vi "Laundry Machine.vi"() -> ()   [LabVIEW 2011]
panel:
  out "1-Rinsing\n2-Washing\n3-Squeezing\n4-Drying":i16[](array[numeric])
  in  "?":bool
  in  "?":bool
  in  "?":bool
  in  "?":bool
  in  "?":bool
  in  "Washing Time(1)":dbl
  in  "Drying Time":dbl
  in  "Squeezing Time":dbl
  in  "Washing Time(2)":dbl
  in  "Rinsing Time":dbl
  in  "Air Temp Variation":dbl
  out "Air Temperature":dbl(slide) scale=0.0..100.0
  out "Air Comp On":bool
  out "Resistor On":bool
  in  "Initial Water Temperature":dbl
  out "Filthy Water":dbl(slide) scale=0.0..10.0
  out "RPM":dbl(knob) scale=0.0..60.0
  out "Mass Flow Rate":dbl(knob) scale=0.0..40.0
  in  "Soap(g)":dbl(slide) scale=0.0..1000.0
  in  "Set Water Temperature":i8(knob) scale=20.0..100.0
  out "Water Temperature(C)":i8(slide) scale=0.0..100.0
  in  "Tank(L)":dbl(slide) scale=0.0..10.0
  in  "Weight":u8
  out "Door Locked":bool
  in  "Lock Door":bool
  in  "Program":i8(knob) scale=0.0..3.0
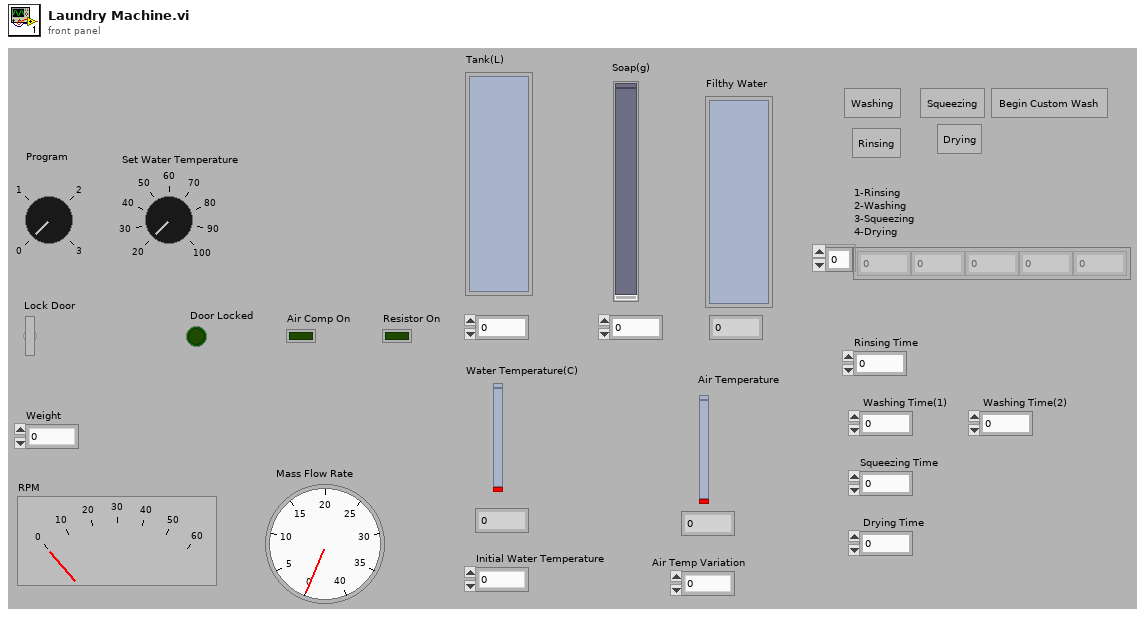
[diagram p1: front panel]
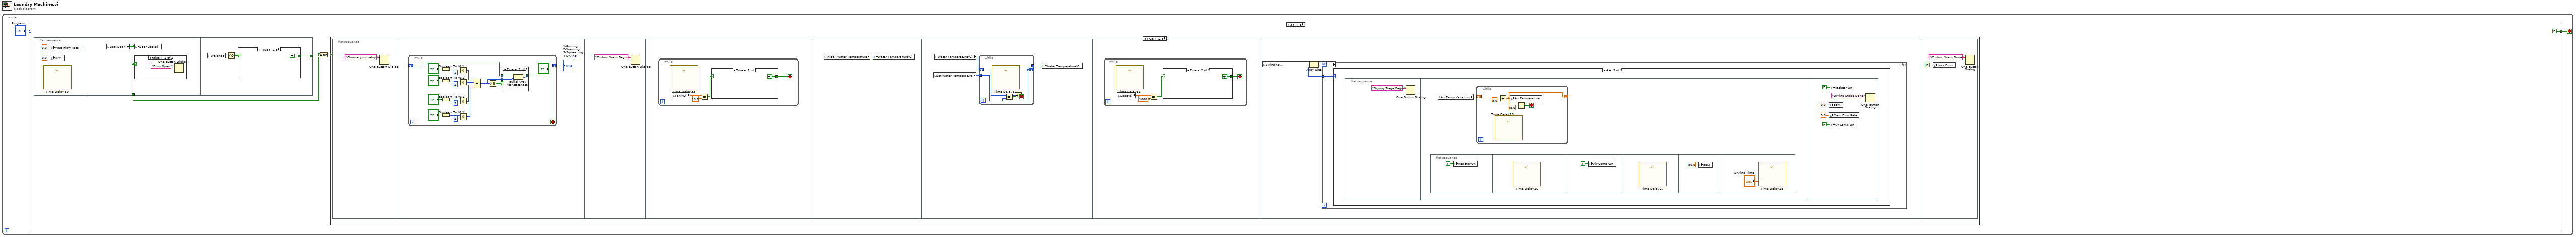
[diagram p0: block diagram]
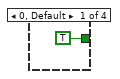
[diagram p2: hidden frame]
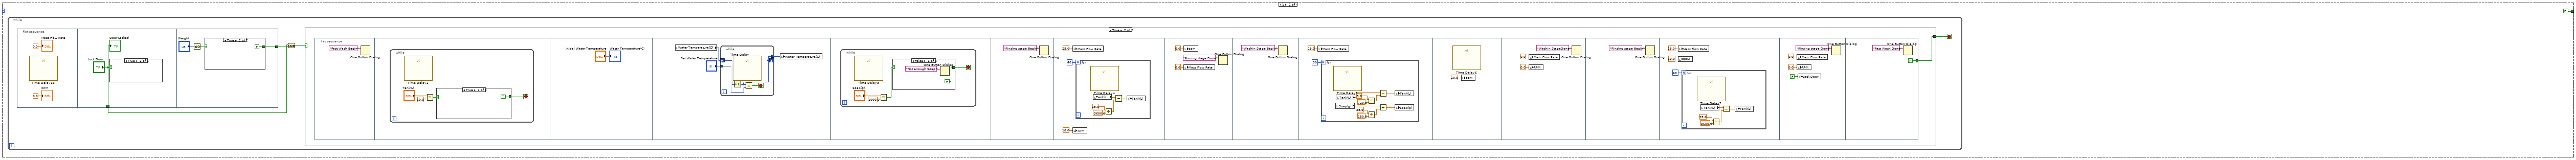
[diagram p3: hidden frame]
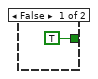
[diagram p4: hidden frame]
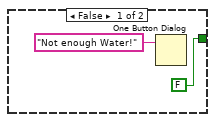
[diagram p5: hidden frame]
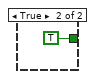
[diagram p6: hidden frame]
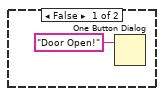
[diagram p7: hidden frame]
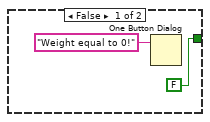
[diagram p8: hidden frame]
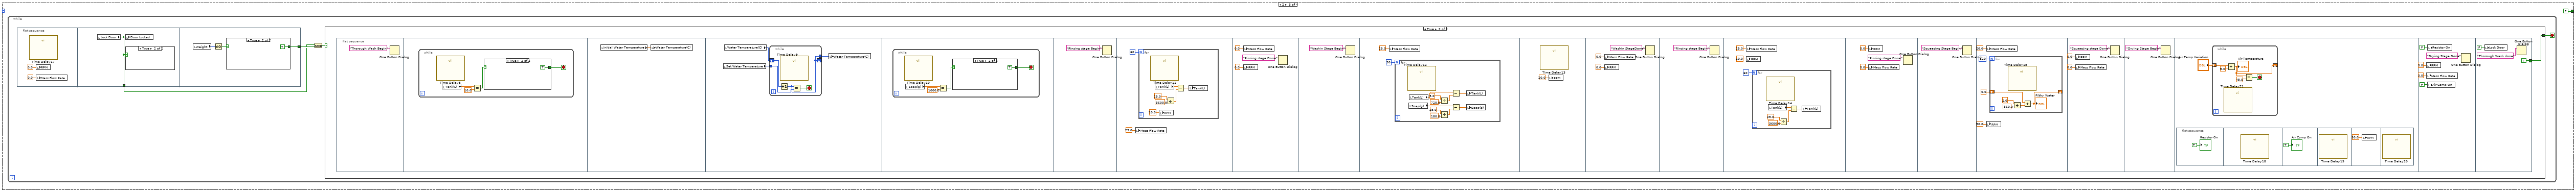
[diagram p9: hidden frame]
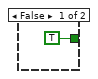
[diagram p10: hidden frame]
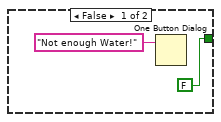
[diagram p11: hidden frame]
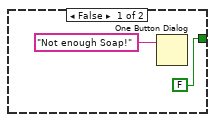
[diagram p12: hidden frame]
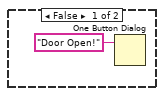
[diagram p13: hidden frame]
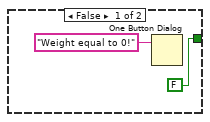
[diagram p14: hidden frame]
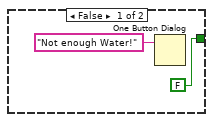
[diagram p17: hidden frame]
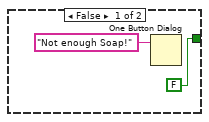
[diagram p18: hidden frame]
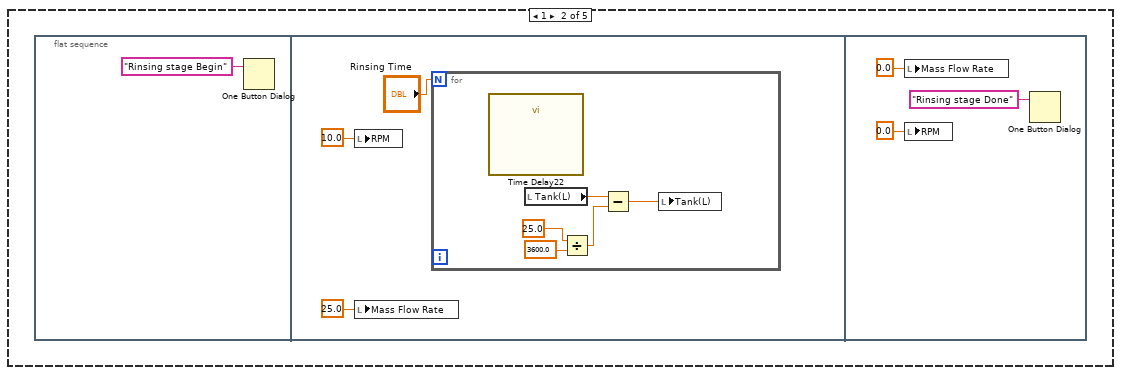
[diagram p20: hidden frame]
diagram:
  n1 = while {
    stop <- w2 stop-if-true
    n2 = case shown="3" "Program" {
      tunnel: [TRUE FALSE FALSE FALSE] -> w2
      frame 0, Default {
      }
      frame 1 {
        n3 = while {
          stop <- w5 stop-if-true
          n4 = flat-sequence {
            tunnel: ["Lock Door"] -> w8
            tunnel: [w82] -> w7
            frame #0 {
              n5 = call "Time Delay16"() -> ()  [unwired: 11 in, 1 out]
              "Mass Flow Rate" <- 0.0 ("Mass Flow Rate")
              "RPM" <- 0.0 ("RPM")
            }
            frame #1 {
              n6 = case shown="True" "Lock Door" {
                frame False {
                  n7 = One Button Dialog(message="Door Open!") -> ()  [unwired: 1 in, 1 out]
                }
                frame True {
                }
              }
              "Door Locked" <- "Lock Door"
            }
            frame #2 {
              n8 = Not Equal To 0?(x="Weight") -> (x != 0?=w83:bool)
              n9 = case shown="True" w83 {
                tunnel: [FALSE TRUE] -> w82
                frame False {
                  n10 = One Button Dialog(message="Weight equal to 0!") -> ()  [unwired: 1 in, 1 out]
                }
                frame True {
                }
              }
            }
          }
          n11 = And(x=w8, y=w7) -> (x .and. y?=w6:bool)
          n12 = case shown="True" w6 {
            tunnel: [TRUE w10] -> w5
            frame False {
            }
            frame True {
              n13 = flat-sequence {
                tunnel: [TRUE] -> w10
                frame #0 {
                  n14 = One Button Dialog(message="Fast Wash Begin" ("Stage")) -> ()  [unwired: 1 in, 1 out]
                }
                frame #1 {
                  n15 = while {
                    stop <- w13 stop-if-true
                    n16 = call "Time Delay2"() -> ()  [unwired: 11 in, 1 out]
                    n17 = Equal?(x="Tank(L)", y=10.0) -> (x = y?=w14:bool)
                    n18 = case shown="True" w14 {
                      tunnel: [FALSE TRUE] -> w13
                      frame False {
                        n19 = One Button Dialog(message="Not enough Water!" ("String 2")) -> ()  [unwired: 1 in, 1 out]
                      }
                      frame True {
                      }
                    }
                  }
                }
                frame #2 {
                  "Water Temperature(C)" <- "Initial Water Temperature"
                }
                frame #3 {
                  n20 = local read "Water Temperature(C)"() -> (w21:i8)
                  n21 = while {
                    tunnel: "Set Water Temperature" -> [w26]
                    shift-right: [w23] -> _
                    shift-left: w21 -> [w24]
                    tunnel: [w23] -> w20
                    stop <- w25 stop-if-true
                    n22 = Increment(x=w24) -> (x+1=w23:i8)
                    n23 = call "Time Delay"() -> ()  [unwired: 11 in, 1 out]
                    n24 = Equal?(x=w23, y=w26) -> (x = y?=w25:bool)
                  }
                  n25 = local write "Water Temperature(C)"(w20) -> ()
                }
                frame #4 {
                  n26 = while {
                    stop <- w28 stop-if-true
                    n27 = call "Time Delay3"() -> ()  [unwired: 11 in, 1 out]
                    n28 = Equal?(x="Soap(g)", y=1000.0) -> (x = y?=w29:bool)
                    n29 = case shown="False" w29 {
                      tunnel: [FALSE TRUE] -> w28
                      frame False {
                        n30 = One Button Dialog(message="Not enough Soap!" ("String 2")) -> ()  [unwired: 1 in, 1 out]
                      }
                      frame True {
                      }
                    }
                  }
                }
                frame #5 {
                  n31 = One Button Dialog(message="Rinsing stage Begin" ("Stage")) -> ()  [unwired: 1 in, 1 out]
                }
                frame #6 {
                  n32 = local write "Mass Flow Rate"(25.0 ("Mass Flow Rate")) -> ()
                  n33 = local write "RPM"(10.0 ("RPM")) -> ()
                  n34 = for {
                    N: 60 -> [_]
                    n35 = call "Time Delay4"() -> ()  [unwired: 11 in, 1 out]
                    n36 = local read "Tank(L)"() -> (w38:dbl)
                    n37 = Divide(x=25.0, y=3600.0) -> (x/y=w40:dbl)
                    n38 = Subtract(x=w38, y=w40) -> (x-y=w39:dbl)
                    n39 = local write "Tank(L)"(w39) -> ()
                  }
                }
                frame #7 {
                  n40 = local write "RPM"(0.0 ("RPM")) -> ()
                  n41 = local write "Mass Flow Rate"(0.0 ("Mass Flow Rate")) -> ()
                  n42 = One Button Dialog(message="Rinsing stage Done" ("Stage")) -> ()  [unwired: 1 in, 1 out]
                }
                frame #8 {
                  n43 = One Button Dialog(message="Washin Stage Begin" ("Stage")) -> ()  [unwired: 1 in, 1 out]
                }
                frame #9 {
                  n44 = local write "Mass Flow Rate"(25.0 ("Mass Flow Rate")) -> ()
                  n45 = for {
                    N: 30 -> [_]
                    n46 = call "Time Delay5"() -> ()  [unwired: 11 in, 1 out]
                    n47 = local read "Soap(g)"() -> (w57:dbl)
                    n48 = local read "Tank(L)"() -> (w50:dbl)
                    n49 = Divide(x=5.0, y=720.0) -> (x/y=w52:dbl)
                    n50 = Divide(x=25.0, y=180.0) -> (x/y=w56:dbl)
                    n51 = Subtract(x=w50, y=w52) -> (x-y=w53:dbl)
                    n52 = Subtract(x=w57, y=w56) -> (x-y=w58:dbl)
                    n53 = local write "Tank(L)"(w53) -> ()
                    n54 = local write "Soap(g)"(w58) -> ()
                  }
                }
                frame #10 {
                  n55 = call "Time Delay6"() -> ()  [unwired: 11 in, 1 out]
                  n56 = local write "RPM"(20.0 ("RPM")) -> ()
                }
                frame #11 {
                  n57 = local write "Mass Flow Rate"(0.0 ("Mass Flow Rate")) -> ()
                  n58 = local write "RPM"(0.0 ("RPM")) -> ()
                  n59 = One Button Dialog(message="Washin StageDone" ("Stage")) -> ()  [unwired: 1 in, 1 out]
                }
                frame #12 {
                  n60 = One Button Dialog(message="Rinsing stage Begin" ("Stage")) -> ()  [unwired: 1 in, 1 out]
                }
                frame #13 {
                  n61 = local write "Mass Flow Rate"(25.0 ("Mass Flow Rate")) -> ()
                  n62 = local write "RPM"(10.0 ("RPM")) -> ()
                  n63 = for {
                    N: 60 -> [_]
                    n64 = call "Time Delay7"() -> ()  [unwired: 11 in, 1 out]
                    n65 = local read "Tank(L)"() -> (w67:dbl)
                    n66 = Divide(x=25.0, y=3600.0) -> (x/y=w69:dbl)
                    n67 = Subtract(x=w67, y=w69) -> (x-y=w68:dbl)
                    n68 = local write "Tank(L)"(w68) -> ()
                  }
                }
                frame #14 {
                  n69 = local write "Mass Flow Rate"(0.0 ("Mass Flow Rate")) -> ()
                  n70 = local write "RPM"(0.0 ("RPM")) -> ()
                  n71 = local write "Lock Door"(FALSE ("Lock Door")) -> ()
                  n72 = One Button Dialog(message="Rinsing stage Done" ("Stage")) -> ()  [unwired: 1 in, 1 out]
                }
                frame #15 {
                  n73 = One Button Dialog(message="Fast Wash Done" ("Stage")) -> ()  [unwired: 1 in, 1 out]
                }
              }
            }
          }
        }
      }
      frame 2 {
        n74 = while {
          stop <- w90 stop-if-true
          n75 = flat-sequence {
            tunnel: [w192] -> w89
            tunnel: [w195] -> w92
            frame #0 {
              n76 = call "Time Delay17"() -> ()  [unwired: 11 in, 1 out]
              n77 = local write "RPM"(0.0 ("RPM")) -> ()
              n78 = local write "Mass Flow Rate"(0.0 ("Mass Flow Rate")) -> ()
            }
            frame #1 {
              n79 = local read "Lock Door"() -> (w192:bool)
              n80 = local write "Door Locked"(w192) -> ()
              n81 = case shown="True" w192 {
                frame False {
                  n82 = One Button Dialog(message="Door Open!") -> ()  [unwired: 1 in, 1 out]
                }
                frame True {
                }
              }
            }
            frame #2 {
              n83 = local read "Weight"() -> (w194:u8)
              n84 = Not Equal To 0?(x=w194) -> (x != 0?=w196:bool)
              n85 = case shown="True" w196 {
                tunnel: [FALSE TRUE] -> w195
                frame False {
                  n86 = One Button Dialog(message="Weight equal to 0!") -> ()  [unwired: 1 in, 1 out]
                }
                frame True {
                }
              }
            }
          }
          n87 = And(x=w89, y=w92) -> (x .and. y?=w91:bool)
          n88 = case shown="True" w91 {
            tunnel: [TRUE w94] -> w90
            frame False {
            }
            frame True {
              n89 = flat-sequence {
                tunnel: [TRUE] -> w94
                frame #0 {
                  n90 = One Button Dialog(message="Thorough Wash Begin" ("Stage")) -> ()  [unwired: 1 in, 1 out]
                }
                frame #1 {
                  n91 = while {
                    stop <- w97 stop-if-true
                    n92 = call "Time Delay8"() -> ()  [unwired: 11 in, 1 out]
                    n93 = local read "Tank(L)"() -> (w96:dbl)
                    n94 = Equal?(x=w96, y=10.0) -> (x = y?=w98:bool)
                    n95 = case shown="True" w98 {
                      tunnel: [FALSE TRUE] -> w97
                      frame False {
                        n96 = One Button Dialog(message="Not enough Water!" ("String 2")) -> ()  [unwired: 1 in, 1 out]
                      }
                      frame True {
                      }
                    }
                  }
                }
                frame #2 {
                  n97 = local read "Initial Water Temperature"() -> (w103:dbl)
                  n98 = local write "Water Temperature(C)"(w103) -> ()
                }
                frame #3 {
                  n99 = local read "Set Water Temperature"() -> (w105:i8)
                  n100 = local read "Water Temperature(C)"() -> (w106:i8)
                  n101 = while {
                    tunnel: w105 -> [w110]
                    shift-right: [w107] -> _
                    shift-left: w106 -> [w108]
                    tunnel: [w107] -> w104
                    stop <- w109 stop-if-true
                    n102 = Increment(x=w108) -> (x+1=w107:i8)
                    n103 = call "Time Delay9"() -> ()  [unwired: 11 in, 1 out]
                    n104 = Equal?(x=w107, y=w110) -> (x = y?=w109:bool)
                  }
                  n105 = local write "Water Temperature(C)"(w104) -> ()
                }
                frame #4 {
                  n106 = while {
                    stop <- w112 stop-if-true
                    n107 = call "Time Delay10"() -> ()  [unwired: 11 in, 1 out]
                    n108 = local read "Soap(g)"() -> (w111:dbl)
                    n109 = Equal?(x=w111, y=1000.0) -> (x = y?=w113:bool)
                    n110 = case shown="True" w113 {
                      tunnel: [FALSE TRUE] -> w112
                      frame False {
                        n111 = One Button Dialog(message="Not enough Soap!" ("String 2")) -> ()  [unwired: 1 in, 1 out]
                      }
                      frame True {
                      }
                    }
                  }
                }
                frame #5 {
                  n112 = One Button Dialog(message="Rinsing stage Begin" ("Stage")) -> ()  [unwired: 1 in, 1 out]
                }
                frame #6 {
                  n113 = local write "Mass Flow Rate"(25.0 ("Mass Flow Rate")) -> ()
                  n114 = for {
                    N: 60 -> [_]
                    n115 = call "Time Delay11"() -> ()  [unwired: 11 in, 1 out]
                    n116 = local read "Tank(L)"() -> (w124:dbl)
                    n117 = local write "RPM"(10.0 ("RPM")) -> ()
                    n118 = Divide(x=25.0, y=3600.0) -> (x/y=w123:dbl)
                    n119 = Subtract(x=w124, y=w123) -> (x-y=w125:dbl)
                    n120 = local write "Tank(L)"(w125) -> ()
                  }
                }
                frame #7 {
                  n121 = local write "Mass Flow Rate"(0.0 ("RPM")) -> ()
                  n122 = local write "RPM"(0.0 ("Mass Flow Rate")) -> ()
                  n123 = One Button Dialog(message="Rinsing stage Done" ("Stage")) -> ()  [unwired: 1 in, 1 out]
                }
                frame #8 {
                  n124 = One Button Dialog(message="Washin Stage Begin" ("Stage")) -> ()  [unwired: 1 in, 1 out]
                }
                frame #9 {
                  n125 = local write "Mass Flow Rate"(25.0 ("Mass Flow Rate")) -> ()
                  n126 = for {
                    N: 30 -> [_]
                    n127 = call "Time Delay12"() -> ()  [unwired: 11 in, 1 out]
                    n128 = local read "Soap(g)"() -> (w139:dbl)
                    n129 = local read "Tank(L)"() -> (w141:dbl)
                    n130 = Divide(x=5.0, y=720.0) -> (x/y=w135:dbl)
                    n131 = Divide(x=25.0, y=180.0) -> (x/y=w138:dbl)
                    n132 = Subtract(x=w141, y=w135) -> (x-y=w142:dbl)
                    n133 = Subtract(x=w139, y=w138) -> (x-y=w140:dbl)
                    n134 = local write "Tank(L)"(w142) -> ()
                    n135 = local write "Soap(g)"(w140) -> ()
                  }
                }
                frame #10 {
                  n136 = call "Time Delay13"() -> ()  [unwired: 11 in, 1 out]
                  n137 = local write "RPM"(20.0 ("RPM")) -> ()
                }
                frame #11 {
                  n138 = local write "Mass Flow Rate"(0.0 ("Mass Flow Rate")) -> ()
                  n139 = local write "RPM"(0.0 ("RPM")) -> ()
                  n140 = One Button Dialog(message="Washin StageDone" ("Stage")) -> ()  [unwired: 1 in, 1 out]
                }
                frame #12 {
                  n141 = One Button Dialog(message="Rinsing stage Begin" ("Stage")) -> ()  [unwired: 1 in, 1 out]
                }
                frame #13 {
                  n142 = local write "Mass Flow Rate"(25.0 ("Mass Flow Rate")) -> ()
                  n143 = local write "RPM"(10.0 ("RPM")) -> ()
                  n144 = for {
                    N: 60 -> [_]
                    n145 = call "Time Delay14"() -> ()  [unwired: 11 in, 1 out]
                    n146 = local read "Tank(L)"() -> (w151:dbl)
                    n147 = Divide(x=25.0, y=3600.0) -> (x/y=w153:dbl)
                    n148 = Subtract(x=w151, y=w153) -> (x-y=w152:dbl)
                    n149 = local write "Tank(L)"(w152) -> ()
                  }
                }
                frame #14 {
                  n150 = local write "RPM"(0.0 ("RPM")) -> ()
                  n151 = local write "Mass Flow Rate"(0.0 ("Mass Flow Rate")) -> ()
                  n152 = One Button Dialog(message="Rinsing stage Done" ("Stage")) -> ()  [unwired: 1 in, 1 out]
                }
                frame #15 {
                  n153 = One Button Dialog(message="Squeezing Stage Begin" ("Stage")) -> ()  [unwired: 1 in, 1 out]
                }
                frame #16 {
                  n154 = local write "Mass Flow Rate"(20.0 ("Mass Flow Rate")) -> ()
                  n155 = local write "RPM"(50.0 ("RPM")) -> ()
                  n156 = for {
                    N: 120 -> [_]
                    shift-right: [w164] -> _
                    shift-left: 0.0 -> [w165]
                    n157 = call "Time Delay15"() -> ()  [unwired: 11 in, 1 out]
                    n158 = Divide(x=2.0, y=360.0) -> (x/y=w166:dbl)
                    n159 = Add(x=w165, y=w166) -> (x+y=w164:dbl)
                    "Filthy Water" <- w164
                  }
                }
                frame #17 {
                  n160 = local write "RPM"(0.0 ("RPM")) -> ()
                  n161 = local write "Mass Flow Rate"(0.0 ("Mass Flow Rate")) -> ()
                  n162 = One Button Dialog(message="Squeezing stage Done" ("Stage")) -> ()  [unwired: 1 in, 1 out]
                }
                frame #18 {
                  n163 = One Button Dialog(message="Drying Stage Begin" ("Stage")) -> ()  [unwired: 1 in, 1 out]
                }
                frame #19 {
                  n164 = flat-sequence {
                    frame #0 {
                      "Resistor On" <- TRUE ("Resistor On")
                    }
                    frame #1 {
                      n165 = call "Time Delay18"() -> ()  [unwired: 11 in, 1 out]
                    }
                    frame #2 {
                      "Air Comp On" <- TRUE ("Air Comp On")
                    }
                    frame #3 {
                      n166 = call "Time Delay19"() -> ()  [unwired: 11 in, 1 out]
                    }
                    frame #4 {
                      n167 = local write "RPM"(50.0 ("RPM")) -> ()
                    }
                    frame #5 {
                      n168 = call "Time Delay20"() -> ()  [unwired: 11 in, 1 out]
                    }
                  }
                  n169 = while {
                    shift-right: [w175] -> _
                    shift-left: "Air Temp Variation" -> [w174]
                    stop <- w176 stop-if-true
                    n170 = call "Time Delay21"() -> ()  [unwired: 11 in, 1 out]
                    n171 = Add(x=w174, y=5.0) -> (x+y=w175:dbl)
                    "Air Temperature" <- w175
                    n172 = Equal?(x=w175, y=45.0) -> (x = y?=w176:bool)
                  }
                }
                frame #20 {
                  n173 = local write "RPM"(0.0 ("RPM")) -> ()
                  n174 = local write "Mass Flow Rate"(0.0 ("Mass Flow Rate")) -> ()
                  n175 = local write "Resistor On"(FALSE ("Resistor On")) -> ()
                  n176 = local write "Air Comp On"(FALSE ("Air Comp On")) -> ()
                  n177 = One Button Dialog(message="Drying Stage Done" ("Stage")) -> ()  [unwired: 1 in, 1 out]
                }
                frame #21 {
                  n178 = local write "Lock Door"(FALSE ("Lock Door")) -> ()
                  n179 = One Button Dialog(message="Thorough Wash done" ("Stage")) -> ()  [unwired: 1 in, 1 out]
                }
              }
            }
          }
        }
      }
      frame 3 {
        n180 = flat-sequence {
          tunnel: [w320] -> w201
          tunnel: [w323] -> w202
          frame #0 {
            n181 = call "Time Delay30"() -> ()  [unwired: 11 in, 1 out]
            n182 = local write "Mass Flow Rate"(0.0 ("Mass Flow Rate")) -> ()
            n183 = local write "RPM"(0.0 ("RPM")) -> ()
          }
          frame #1 {
            n184 = local read "Lock Door"() -> (w320:bool)
            n185 = local write "Door Locked"(w320) -> ()
            n186 = case shown="False" w320 {
              frame False {
                n187 = One Button Dialog(message="Door Open!") -> ()  [unwired: 1 in, 1 out]
              }
              frame True {
              }
            }
          }
          frame #2 {
            n188 = local read "Weight"() -> (w322:u8)
            n189 = Not Equal To 0?(x=w322) -> (x != 0?=w324:bool)
            n190 = case shown="True" w324 {
              tunnel: [FALSE TRUE] -> w323
              frame False {
                n191 = One Button Dialog(message="Weight equal to 0!") -> ()  [unwired: 1 in, 1 out]
              }
              frame True {
              }
            }
          }
        }
        n192 = And(x=w201, y=w202) -> (x .and. y?=w200:bool)
        n193 = case shown="True" w200 {
          frame False {
          }
          frame True {
            n194 = flat-sequence {
              frame #0 {
                n195 = One Button Dialog(message="Choose your setup" ("Stage")) -> ()  [unwired: 1 in, 1 out]
              }
              frame #1 {
                n196 = while {
                  shift-right: [w208] -> w205
                  shift-left: _ -> [w206]
                  stop <- "?" stop-if-true
                  n197 = Boolean To (0,1)(Boolean="?") -> (0, 1=w221:i16)
                  n198 = Boolean To (0,1)(Boolean="?") -> (0, 1=w218:i16)
                  n199 = Boolean To (0,1)(Boolean="?") -> (0, 1=w220:i16)
                  n200 = Boolean To (0,1)(Boolean="?") -> (0, 1=w219:i16)
                  n201 = Multiply(x=w221, y=i16 1) -> (x*y=w213:i16)
                  n202 = Multiply(x=w218, y=i16 2) -> (x*y=w212:i16)
                  n203 = Multiply(x=w220, y=i16 3) -> (x*y=w211:i16)
                  n204 = Multiply(x=w219, y=i16 4) -> (x*y=w210:i16)
                  n205 = Compound Arithmetic op=ADD(w213, w212, w211, w210) -> (w207:i16)
                  n206 = Not Equal To 0?(x=w207) -> (x != 0?=w209:bool)
                  n207 = case shown="True" w209 {
                    tunnel: [w227 w230] -> w208
                    tunnel: w207 -> [_ w229]
                    tunnel: w206 -> [w227 w228]
                    frame False {
                    }
                    frame True {
                      n208 = Build Array (concatenate)(w228, w229) -> (w230:i16[])
                    }
                  }
                }
                "1-Rinsing\n2-Washing\n3-Squeezing\n4-Drying" <- w205
              }
              frame #2 {
                n209 = One Button Dialog(message="Custom Wash Begin" ("Stage")) -> ()  [unwired: 1 in, 1 out]
              }
              frame #3 {
                n210 = while {
                  stop <- w233 stop-if-true
                  n211 = call "Time Delay33"() -> ()  [unwired: 11 in, 1 out]
                  n212 = local read "Tank(L)"() -> (w232:dbl)
                  n213 = Equal?(x=w232, y=10.0) -> (x = y?=w234:bool)
                  n214 = case shown="True" w234 {
                    tunnel: [FALSE TRUE] -> w233
                    frame False {
                      n215 = One Button Dialog(message="Not enough Water!" ("String 2")) -> ()  [unwired: 1 in, 1 out]
                    }
                    frame True {
                    }
                  }
                }
              }
              frame #4 {
                n216 = local read "Initial Water Temperature"() -> (w239:dbl)
                n217 = local write "Water Temperature(C)"(w239) -> ()
              }
              frame #5 {
                n218 = local read "Set Water Temperature"() -> (w241:i8)
                n219 = local read "Water Temperature(C)"() -> (w240:i8)
                n220 = while {
                  tunnel: w241 -> [w246]
                  shift-right: [w243] -> _
                  shift-left: w240 -> [w244]
                  tunnel: [w243] -> w242
                  stop <- w245 stop-if-true
                  n221 = call "Time Delay32"() -> ()  [unwired: 11 in, 1 out]
                  n222 = Increment(x=w244) -> (x+1=w243:i8)
                  n223 = Equal?(x=w243, y=w246) -> (x = y?=w245:bool)
                }
                n224 = local write "Water Temperature(C)"(w242) -> ()
              }
              frame #6 {
                n225 = while {
                  stop <- w248 stop-if-true
                  n226 = call "Time Delay31"() -> ()  [unwired: 11 in, 1 out]
                  n227 = local read "Soap(g)"() -> (w247:dbl)
                  n228 = Equal?(x=w247, y=1000.0) -> (x = y?=w249:bool)
                  n229 = case shown="True" w249 {
                    tunnel: [FALSE TRUE] -> w248
                    frame False {
                      n230 = One Button Dialog(message="Not enough Soap!" ("String 2")) -> ()  [unwired: 1 in, 1 out]
                    }
                    frame True {
                    }
                  }
                }
              }
              frame #7 {
                n231 = local read "1-Rinsing\n2-Washing\n3-Squeezing\n4-Drying"() -> (w254:i16[])
                n232 = Array Size(array=w254) -> (size(s)=w255:i32)
                n233 = for {
                  N: w255 -> [_]
                  tunnel: w254 -> [w256] mode=indexing
                  n234 = case shown="4" w256 {
                    frame 0, Default {
                    }
                    frame 1 {
                      n235 = flat-sequence {
                        frame #0 {
                          n236 = One Button Dialog(message="Rinsing stage Begin" ("Stage")) -> ()  [unwired: 1 in, 1 out]
                        }
                        frame #1 {
                          n237 = local write "RPM"(10.0 ("RPM")) -> ()
                          n238 = local write "Mass Flow Rate"(25.0 ("Mass Flow Rate")) -> ()
                          n239 = for {
                            N: "Rinsing Time" -> [_]
                            n240 = call "Time Delay22"() -> ()  [unwired: 11 in, 1 out]
                            n241 = local read "Tank(L)"() -> (w264:dbl)
                            n242 = Divide(x=25.0, y=3600.0) -> (x/y=w263:dbl)
                            n243 = Subtract(x=w264, y=w263) -> (x-y=w265:dbl)
                            n244 = local write "Tank(L)"(w265) -> ()
                          }
                        }
                        frame #2 {
                          n245 = local write "Mass Flow Rate"(0.0 ("RPM")) -> ()
                          n246 = local write "RPM"(0.0 ("Mass Flow Rate")) -> ()
                          n247 = One Button Dialog(message="Rinsing stage Done" ("Stage")) -> ()  [unwired: 1 in, 1 out]
                        }
                      }
                    }
                    frame 2 {
                      n248 = flat-sequence {
                        frame #0 {
                          n249 = One Button Dialog(message="Washin Stage Begin" ("Stage")) -> ()  [unwired: 1 in, 1 out]
                        }
                        frame #1 {
                          n250 = local write "Mass Flow Rate"(25.0 ("Mass Flow Rate")) -> ()
                          n251 = for {
                            N: "Washing Time(1)" -> [_]
                            n252 = call "Time Delay24"() -> ()  [unwired: 11 in, 1 out]
                            n253 = local read "Soap(g)"() -> (w278:dbl)
                            n254 = local read "Tank(L)"() -> (w280:dbl)
                            n255 = Divide(x=5.0, y=720.0) -> (x/y=w274:dbl)
                            n256 = Divide(x=25.0, y=180.0) -> (x/y=w277:dbl)
                            n257 = Subtract(x=w280, y=w274) -> (x-y=w281:dbl)
                            n258 = Subtract(x=w278, y=w277) -> (x-y=w279:dbl)
                            n259 = local write "Tank(L)"(w281) -> ()
                            n260 = local write "Soap(g)"(w279) -> ()
                          }
                        }
                        frame #2 {
                          n261 = local write "RPM"(20.0 ("RPM")) -> ()
                          n262 = call "Time Delay23"("Delay Time (s)"="Washing Time(2)") -> ()  [unwired: 10 in, 1 out]
                        }
                        frame #3 {
                          n263 = local write "Mass Flow Rate"(0.0 ("Mass Flow Rate")) -> ()
                          n264 = local write "RPM"(0.0 ("RPM")) -> ()
                          n265 = One Button Dialog(message="Washin StageDone" ("Stage")) -> ()  [unwired: 1 in, 1 out]
                        }
                      }
                    }
                    frame 3 {
                      n266 = flat-sequence {
                        frame #0 {
                          n267 = One Button Dialog(message="Squeezing Stage Begin" ("Stage")) -> ()  [unwired: 1 in, 1 out]
                        }
                        frame #1 {
                          n268 = local write "Mass Flow Rate"(20.0 ("Mass Flow Rate")) -> ()
                          n269 = local write "RPM"(50.0 ("RPM")) -> ()
                          n270 = for {
                            N: "Squeezing Time" -> [_]
                            shift-right: [w292] -> _
                            shift-left: 0.0 -> [w293]
                            n271 = call "Time Delay25"() -> ()  [unwired: 11 in, 1 out]
                            n272 = Divide(x=2.0, y=360.0) -> (x/y=w294:dbl)
                            n273 = Add(x=w293, y=w294) -> (x+y=w292:dbl)
                            n274 = local write "Filthy Water"(w292) -> ()
                          }
                        }
                        frame #2 {
                          n275 = local write "RPM"(0.0 ("RPM")) -> ()
                          n276 = local write "Mass Flow Rate"(0.0 ("Mass Flow Rate")) -> ()
                          n277 = One Button Dialog(message="Squeezing stage Done" ("Stage")) -> ()  [unwired: 1 in, 1 out]
                        }
                      }
                    }
                    frame 4 {
                      n278 = flat-sequence {
                        frame #0 {
                          n279 = One Button Dialog(message="Drying Stage Begin" ("Stage")) -> ()  [unwired: 1 in, 1 out]
                        }
                        frame #1 {
                          n280 = flat-sequence {
                            frame #0 {
                              n281 = local write "Resistor On"(TRUE ("Resistor On")) -> ()
                            }
                            frame #1 {
                              n282 = call "Time Delay26"() -> ()  [unwired: 11 in, 1 out]
                            }
                            frame #2 {
                              n283 = local write "Air Comp On"(TRUE ("Air Comp On")) -> ()
                            }
                            frame #3 {
                              n284 = call "Time Delay27"() -> ()  [unwired: 11 in, 1 out]
                            }
                            frame #4 {
                              n285 = local write "RPM"(50.0 ("RPM")) -> ()
                            }
                            frame #5 {
                              n286 = call "Time Delay28"("Delay Time (s)"="Drying Time") -> ()  [unwired: 10 in, 1 out]
                            }
                          }
                          n287 = local read "Air Temp Variation"() -> (w301:dbl)
                          n288 = while {
                            shift-right: [w302] -> _
                            shift-left: w301 -> [w303]
                            stop <- w304 stop-if-true
                            n289 = call "Time Delay29"() -> ()  [unwired: 11 in, 1 out]
                            n290 = Add(x=w303, y=5.0) -> (x+y=w302:dbl)
                            n291 = local write "Air Temperature"(w302) -> ()
                            n292 = Equal?(x=w302, y=45.0) -> (x = y?=w304:bool)
                          }
                        }
                        frame #2 {
                          n293 = local write "RPM"(0.0 ("RPM")) -> ()
                          n294 = local write "Mass Flow Rate"(0.0 ("Mass Flow Rate")) -> ()
                          n295 = local write "Resistor On"(FALSE ("Resistor On")) -> ()
                          n296 = local write "Air Comp On"(FALSE ("Air Comp On")) -> ()
                          n297 = One Button Dialog(message="Drying Stage Done" ("Stage")) -> ()  [unwired: 1 in, 1 out]
                        }
                      }
                    }
                  }
                }
              }
              frame #8 {
                n298 = local write "Lock Door"(FALSE ("Door Locked")) -> ()
                n299 = One Button Dialog(message="Custom Wash Done" ("Stage")) -> ()  [unwired: 1 in, 1 out]
              }
            }
          }
        }
      }
    }
  }
